vi "Read ESTTL Setup.vi"(8 "error in (no error)":errorcluster, 11 "DCM-DSI-HW in":refnum<class "DCM-DSI.lvclass">) -> (0 "error out":errorcluster, 2 "DiffIO ESTTL":T1[](array[typedef]) {"Skip Fire Index" max=7; "Angles"."Duration [s]" format="%#_3p"; "Frequency [Hz]" format="%#_3p"}, 3 "DCM-DSI-HW out":refnum<class "DCM-DSI.lvclass">)   [LabVIEW 2016, in "DCM-DSI.lvclass"]
uses:
  DCM-DSI.lvclass
  <vilib>/Powertrain Controls/Device Drivers/DCM/ESTTL/RT/Setup.ctl
  <vilib>/Powertrain Controls/Device Drivers/DCM/ESTTL/FPGA/Mode.ctl
  <vilib>/Powertrain Controls/Device Drivers/DCM/ESTTL/RT/Angle Control.ctl
  DCM-DSI.lvclass/DCM-DSI.ctl
  <vilib>/Powertrain Controls/Device Drivers/DCM/ESTTL/FPGA/DCM - FPGA - ESTTL.lvlib
  <vilib>/Powertrain Controls/Device Drivers/DCM/ESTTL/RT/DCM - RT - ESTTL.lvlib
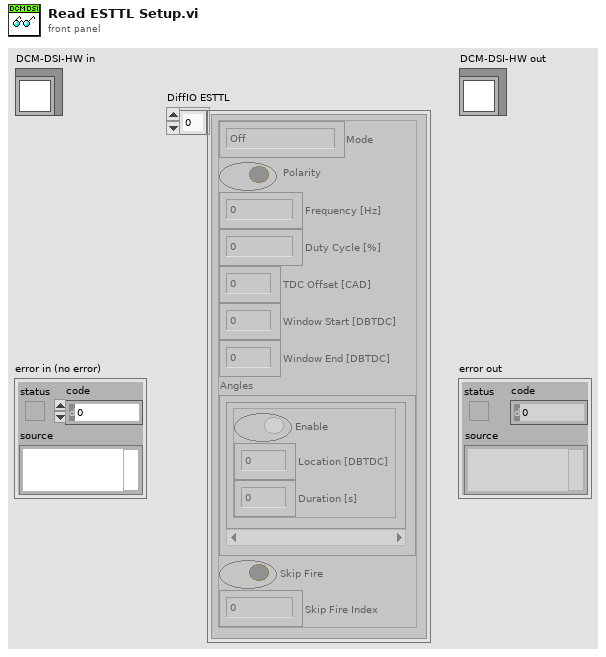
[diagram p1: front panel]
types:
  T1 = typedef "DCM - RT - ESTTL.lvlib/Setup.ctl" = cluster{"Mode":T2, "Polarity":bool, "Frequency [Hz]":sgl, "Duty Cycle [%]":sgl, "TDC Offset [CAD]":sgl, "Window Start [DBTDC]":sgl, "Window End [DBTDC]":sgl, "Angles":T3[], "Skip Fire":bool, "Skip Fire Index":u8}
  T2 = typedef "DCM - FPGA - ESTTL.lvlib/Mode.ctl" = enum8{"Off", "Pulse Width Modulation", "Engine Position Tracking"}
  T3 = typedef "DCM - RT - ESTTL.lvlib/Angle Control.ctl" = cluster{"Enable":bool, "Location [DBTDC]":sgl, "Duration [s]":sgl}
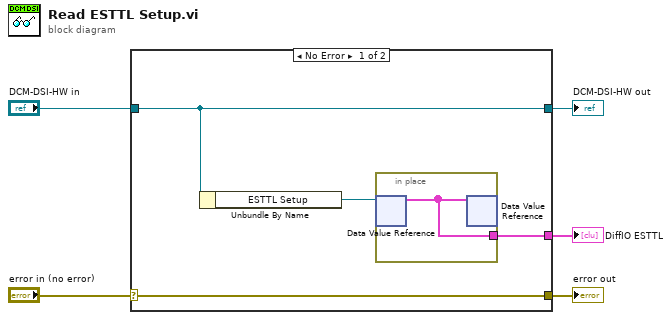
[diagram p0: block diagram]
diagram:
  n1 = case shown="No Error" "error in (no error)" {
    selector: "error in (no error)" -> [w9 w12]
    tunnel: [w9 w12] -> w4
    tunnel: [w7 w11] -> w2
    tunnel: "DCM-DSI-HW in" -> [w7 w11]
    tunnel: [w6 _] -> w1
    frame No Error {
      n2 = Unbundle By Name(w7) -> ("ESTTL Setup"=w8:refnum<data-value>)
      n3 = in-place {
        in-place-border: [w10] -> w6
        n4 = in-place-dvr #1(w8) -> (w10:T1[])  [unwired: 1 out]
        n5 = in-place-dvr #1(w10) -> ()  [unwired: 2 out]
      }
    }
    frame Error {
    }
  }
  "error out" <- w4
  "DCM-DSI-HW out" <- w2
  "DiffIO ESTTL" <- w1
